vi "setSerializedData.vi"(0 "reference":refnum<class "PointNode.lvclass">, 1 "parent":refnum<class "AbstractNode.lvclass">, 2 "children":refnum<class "AbstractNode.lvclass">[](array[class]), 3 "xmlOut":string, 5 "error in (no error)":errorcluster) -> (14 "reference out":refnum<class "PointNode.lvclass">, 19 "error out":errorcluster)   [LabVIEW 2016, in "PointNode.lvclass"]
doc: "setSerializedData"
uses:
  <resource>/Framework/Providers/Open_GDS/UML/PointNode_class/PointNode.lvclass
  C:/Program Files (x86)/National Instruments/LabVIEW 2016/resource/Framework/Providers/Open_GDS/UML/AbstractNode_class/AbstractNode.lvclass
  <resource>/Framework/Providers/Open_GDS/UML/AbstractNode_class/AbstractNode.lvclass
  <resource>/Framework/Providers/Open_GDS/UML/General/Point/Point Point2D.ctl
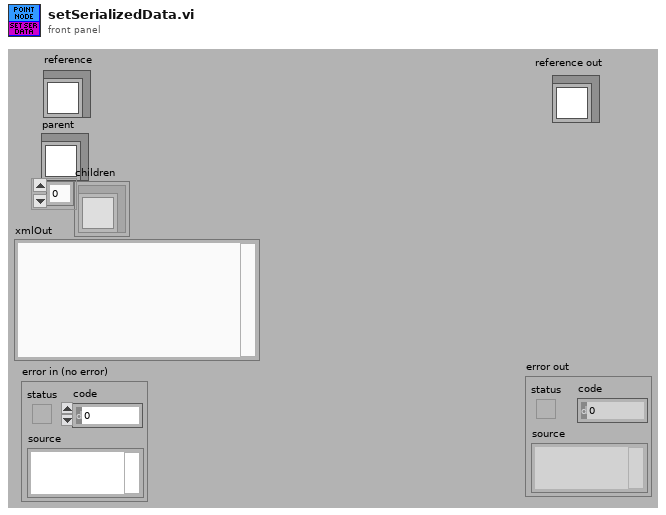
[diagram p1: front panel]
types:
  T1 = typedef "Point Point2D.ctl" = cluster{"x":dbl, "y":dbl}
  T2 = cluster{"Base class":cluster{"parent":refnum<k1>, "children":refnum<k1>[]}, "point":T1}
  T3 = typedef "PointNode.lvclass/ObjectAttributes.ctl" = cluster{"point":T1}
  T4 = typedef "AbstractNode.lvclass/ObjectAttributes.ctl" = cluster{"parent":refnum<class "AbstractNode.lvclass">, "children":refnum<class "AbstractNode.lvclass">[], "Hidden":bool}
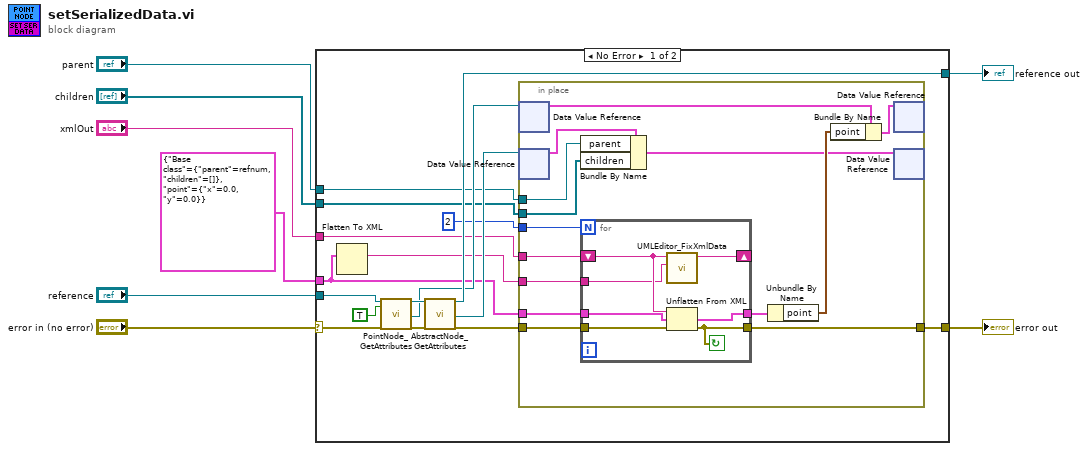
[diagram p0: block diagram]
diagram:
  n1 = case shown="No Error" "error in (no error)" {
    selector: "error in (no error)" -> [w24 w46]
    tunnel: "reference" -> [w23 w47]
    tunnel: [w11 w46] -> w6
    tunnel: [w22 w47] -> w5
    tunnel: "xmlOut" -> [w13 _]
    tunnel: "parent" -> [w10 _]
    tunnel: "children" -> [w9 _]
    tunnel: T2 {"Base class"={"parent"=refnum, "children"=[]}, "point"={"x"=0.0, "y"=0.0}} ("Attributes") -> [w14 _]
    frame No Error {
      n2 = Flatten To XML(anything=w14) -> (xml string=w12:string)
      n3 = call <resource>:"PointNode_GetAttributes.vi"("reference in"=w23, "OnlyGetDvrReference(False)"=TRUE, "error in (no error)"=w24) -> ("reference out"=w20:refnum<class "PointNode.lvclass">, "DataRef"=w18:refnum<data-value>, "error out"=w19:errorcluster)  [unwired: 13 in, 1 out]
      n4 = call <resource>:"AbstractNode_GetAttributes.vi"("reference in"=w20, "error in (no error)"=w19) -> ("reference out"=w22:refnum<class "PointNode.lvclass">, "DataRef"=w17:refnum<data-value>, "error out"=w15:errorcluster)  [unwired: 14 in, 1 out]
      n5 = in-place {
        in-place-border: 2 -> [w34]
        in-place-border: w15 -> [w33]
        in-place-border: w14 -> [w32]
        in-place-border: w13 -> [w31]
        in-place-border: w12 -> [w30]
        in-place-border: [w29] -> w11
        in-place-border: w10 -> [w27]
        in-place-border: w9 -> [w26]
        n6 = in-place-dvr #1(w18) -> (w38:T3)  [unwired: 1 out]
        n7 = in-place-dvr #2(w17) -> (w28:T4)  [unwired: 1 out]
        n8 = Bundle By Name(cluster=w28, "parent"=w27, "children"=w26) -> (w25:T4)
        n9 = for {
          N: w34 -> [_]
          tunnel: w33 -> [w45]
          tunnel: [w42] -> w29
          tunnel: [w44] -> w35
          tunnel: w32 -> [w43]
          shift-right: [w41] -> _
          shift-left: w31 -> [w40]
          tunnel: w30 -> [w39]
          stop <- w42 continue-if-true
          n10 = call <resource>:"UMLEditor_FixXmlData.vi"("XmlTemplateIn"=w39, "xmlIn"=w40) -> ("XML OUt"=w41:string)  [unwired: 9 in]
          n11 = Unflatten From XML(xml string=w40, type=w43, error in (no error)=w45) -> (value=w44:T2, error out=w42:errorcluster)
        }
        n12 = Unbundle By Name(w35) -> ("point"=w37:T1)
        n13 = Bundle By Name(cluster=w38, "point"=w37) -> (w36:T3)
        n14 = in-place-dvr #1(w36) -> ()  [unwired: 2 out]
        n15 = in-place-dvr #2(w25) -> ()  [unwired: 2 out]
      }
    }
    frame Error {
    }
  }
  "reference out" <- w5
  "error out" <- w6
